vi "worksheet set zoom.vi"(8 "error in (no error)":errorcluster, 10 "scale":u16, 11 "worksheet":u32) -> (0 "error out":errorcluster)   [LabVIEW 8.6]
doc: "void worksheet_set_zoom(lxw_worksheet worksheet, uint16_t scale);"
uses:
  pending_lvxlsxwriter/xlsxwriter.dll
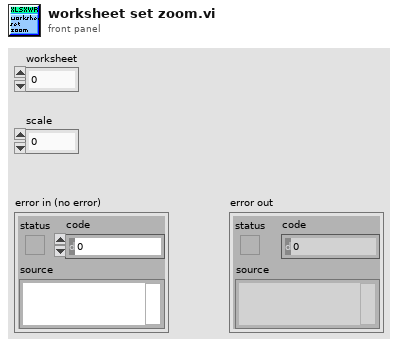
[diagram p1: front panel]
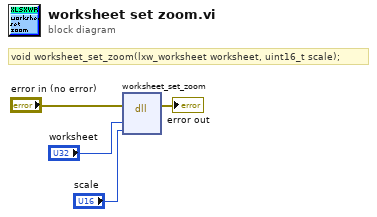
[diagram p0: block diagram]
diagram:
  # "void worksheet_set_zoom(lxw_worksheet worksheet, uint16_t scale);"
  n1 = dll-call lib="C:/Users/WDAGUtilityAccount/Desktop/pending_lvxlsxwriter/xlsxwriter.*" fn="worksheet_set_zoom"(error in="error in (no error)", "worksheet"="worksheet", "scale"="scale") -> (error out=→"error out":errorcluster)  [unwired: 5 in, 1 out]
